vi "关键参数交互.vi"(9 "量程选择":enum16{"低量程", "高量程"}(ring), 11 "模型":enum32{"线性", "多项式", "折线"}(ring)) -> ()   [LabVIEW 2016, in "斯坦道CODMn.lvlib"]
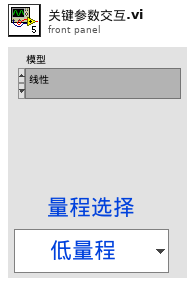
[diagram p1: front panel]
types:
  T1 = cluster{"chose":string, "公式":cluster{"X^2":dbl, "X":dbl, "b":dbl}}
  T2 = cluster{"测量量程":dbl, "测量精度":dbl, "测量间隔":dbl, "消解温度":dbl, "消解时长":dbl, "空白校准时间":timestamp, "曲线截距":dbl, "曲线斜率":dbl, "测量检出限":dbl, "测量信号值":dbl, "线性相关系数":dbl, "二次多项式系数":dbl, "标样校准时间":timestamp, "稀释倍数":dbl, "三项式系数":dbl, "空白标定系数":dbl, "量程系数":dbl, "F0/ORPA":dbl, "F1/ORPB":dbl, "F2/ORPK":dbl, "F3":dbl, "F4":dbl, "F5":dbl, "F6":dbl, "F7":dbl, "X0/滴定数":dbl, "量程":dbl}
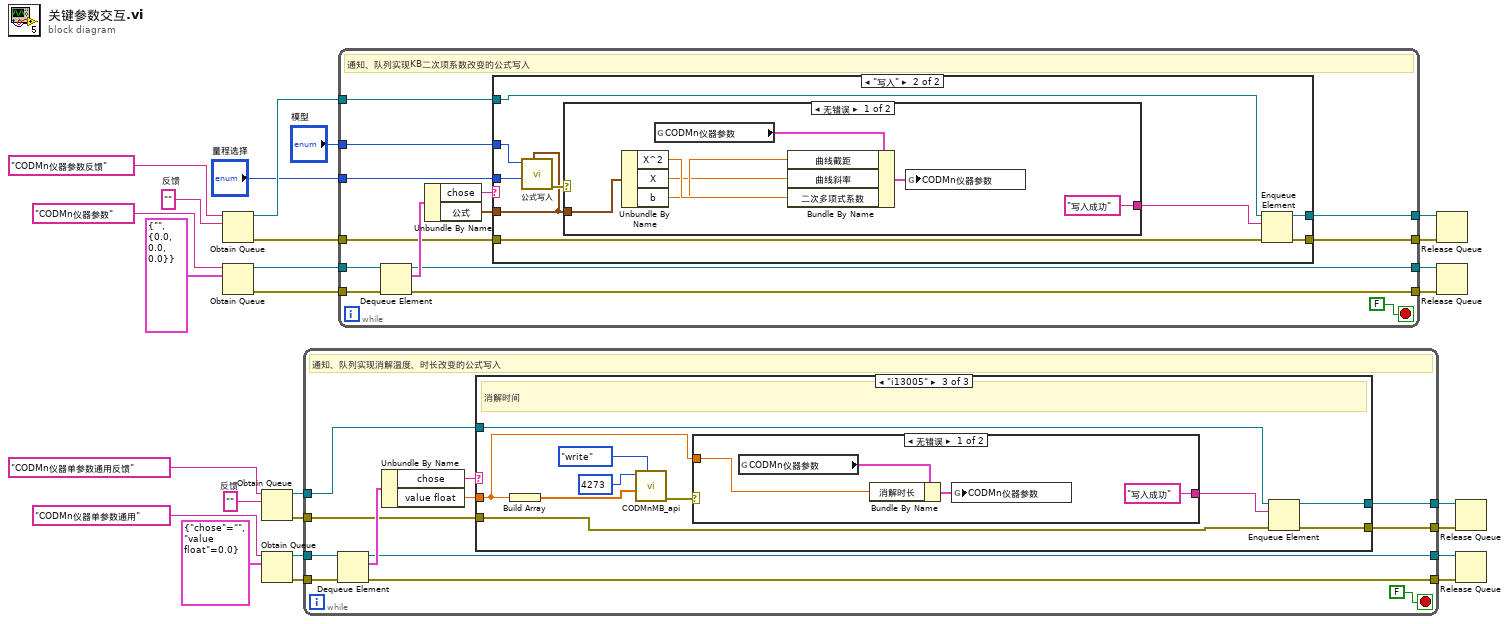
[diagram p0: block diagram]
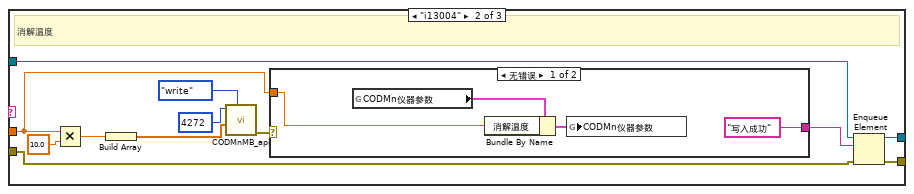
[diagram p3: hidden frame]
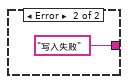
[diagram p4: hidden frame]
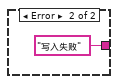
[diagram p5: hidden frame]
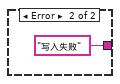
[diagram p7: hidden frame]
diagram:
  w9 = ""  # 反馈
  w18 = ""  # 反馈
  n1 = Obtain Queue(name (unnamed)="CODMn仪器参数反馈" ("名称（未命名）"), element data type=w18) -> (queue out=w19:refnum<queue>, error out=w17:errorcluster)  [unwired: 3 in, 1 out]
  n2 = Obtain Queue(name (unnamed)="CODMn仪器参数" ("名称（未命名）"), element data type=T1 {"chose"="", "公式"={"X^2"=0.0, "X"=0.0, "b"=0.0}}) -> (queue out=w26:refnum<queue>, error out=w25:errorcluster)  [unwired: 3 in, 1 out]
  n3 = Obtain Queue(name (unnamed)="CODMn仪器单参数通用反馈" ("名称（未命名）"), element data type=w9) -> (queue out=w8:refnum<queue>, error out=w10:errorcluster)  [unwired: 3 in, 1 out]
  n4 = Obtain Queue(name (unnamed)="CODMn仪器单参数通用" ("名称（未命名）"), element data type=cluster{"chose":string, "value float":dbl} {"chose"="", "value float"=0.0}) -> (queue out=w1:refnum<queue>, error out=w2:errorcluster)  [unwired: 3 in, 1 out]
  n5 = while {
    tunnel: w1 -> [w37]
    tunnel: w2 -> [w36]
    tunnel: [w32] -> w5
    tunnel: [w31] -> w6
    tunnel: w8 -> [w30]
    tunnel: w10 -> [w29]
    tunnel: [w28] -> w11
    tunnel: [w27] -> w12
    stop <- FALSE stop-if-true
    # "通知、队列实现消解温度、时长改变的公式写入"
    n6 = Dequeue Element(queue=w37, error in (no error)=w36) -> (queue out=w32:refnum<queue>, element=w35:cluster{"chose":string, "value float":dbl}, error out=w31:errorcluster)  [unwired: 1 in, 1 out]
    n7 = Unbundle By Name(w35) -> ("chose"=w34:string, "value float"=w33:dbl)
    n8 = case shown="\"i13005\"" w34 {
      tunnel: w33 -> [_ w41 w58]
      tunnel: w30 -> [w40 w52 w67]
      tunnel: w29 -> [w39 w50 w63]
      tunnel: [w40 w49 w65] -> w28
      tunnel: [w39 w48 w64] -> w27
      frame "假", Default {
      }
      frame "i13004" {
        # "消解温度"
        n9 = Multiply(x=w41, y=10.0) -> (x*y=w44:dbl)
        n10 = Build Array(w44) -> (w43:dbl[])
        n11 = call "CODMnMB_api.vi"("STEP"=enum16{"open", "read", "write", "close"}."write", "values"=w43, "starting address"=u16 4272) -> ("error out"=w42:errorcluster)  [unwired: 6 in, 2 out]
        n12 = case shown="无错误" w42 {
          tunnel: ["写入成功" ("消息") "写入失败" ("消息")] -> w51
          tunnel: w41 -> [w53 _]
          frame No Error {
            n13 = global read "CODMn断电保存全局变量.vi" "CODMn仪器参数"() -> (w55:T2)
            n14 = Bundle By Name(cluster=w55, "消解温度"=w53) -> (w54:T2)
            n15 = global write "CODMn断电保存全局变量.vi" "CODMn仪器参数"(w54) -> ()
          }
          frame Error {
          }
        }
        n16 = Enqueue Element(queue=w52, element=w51, error in (no error)=w50) -> (queue out=w49:refnum<queue>, error out=w48:errorcluster)  [unwired: 1 in, 1 out]
      }
      frame "i13005" {
        # "消解时间"
        n17 = Build Array(w58) -> (w60:dbl[])
        n18 = call "CODMnMB_api.vi"("STEP"=enum16{"open", "read", "write", "close"}."write", "values"=w60, "starting address"=u16 4273) -> ("error out"=w59:errorcluster)  [unwired: 6 in, 2 out]
        n19 = case shown="无错误" w59 {
          tunnel: ["写入成功" ("消息") "写入失败" ("消息")] -> w66
          tunnel: w58 -> [w69 _]
          frame No Error {
            n20 = global read "CODMn断电保存全局变量.vi" "CODMn仪器参数"() -> (w70:T2)
            n21 = Bundle By Name(cluster=w70, "消解时长"=w69) -> (w68:T2)
            n22 = global write "CODMn断电保存全局变量.vi" "CODMn仪器参数"(w68) -> ()
          }
          frame Error {
          }
        }
        n23 = Enqueue Element(queue=w67, element=w66, error in (no error)=w63) -> (queue out=w65:refnum<queue>, error out=w64:errorcluster)  [unwired: 1 in, 1 out]
      }
    }
  }
  n24 = while {
    tunnel: w26 -> [w85]
    tunnel: w25 -> [w84]
    tunnel: [w80] -> w22
    tunnel: [w79] -> w21
    tunnel: w19 -> [w78]
    tunnel: w17 -> [w77]
    tunnel: [w76] -> w16
    tunnel: [w75] -> w15
    tunnel: "模型" -> [w74]
    tunnel: "量程选择" -> [w73]
    stop <- FALSE stop-if-true
    # "通知、队列实现KB二次项系数改变的公式写入"
    n25 = Dequeue Element(queue=w85, error in (no error)=w84) -> (queue out=w80:refnum<queue>, element=w83:T1, error out=w79:errorcluster)  [unwired: 1 in, 1 out]
    n26 = Unbundle By Name(w83) -> ("chose"=w82:string, "公式"=w81:cluster{"X^2":dbl, "X":dbl, "b":dbl})
    n27 = case shown="\"写入\"" w82 {
      tunnel: w81 -> [_ w90]
      tunnel: w78 -> [w88 w97]
      tunnel: w77 -> [w87 w95]
      tunnel: [w88 w94] -> w76
      tunnel: [w87 w93] -> w75
      tunnel: w74 -> [_ w91]
      tunnel: w73 -> [_ w89]
      frame "假", Default {
      }
      frame "写入" {
        n28 = call "公式写入.vi"("公式"=w90, "量程选择"=w89, "模型"=w91) -> ("error out"=w92:errorcluster)  [unwired: 8 in]
        n29 = case shown="无错误" w92 {
          tunnel: ["写入成功" ("消息") "写入失败" ("消息")] -> w96
          tunnel: w90 -> [w98 _]
          frame No Error {
            n30 = Unbundle By Name(w98) -> ("X^2"=w101:dbl, "X"=w99:dbl, "b"=w100:dbl)
            n31 = global read "CODMn断电保存全局变量.vi" "CODMn仪器参数"() -> (w102:T2)
            n32 = Bundle By Name(cluster=w102, "曲线截距"=w100, "曲线斜率"=w99, "二次多项式系数"=w101) -> (w103:T2)
            n33 = global write "CODMn断电保存全局变量.vi" "CODMn仪器参数"(w103) -> ()
          }
          frame Error {
          }
        }
        n34 = Enqueue Element(queue=w97, element=w96, error in (no error)=w95) -> (queue out=w94:refnum<queue>, error out=w93:errorcluster)  [unwired: 1 in, 1 out]
      }
    }
  }
  n35 = Release Queue(queue=w16, error in (no error)=w15) -> ()  [unwired: 1 in, 3 out]
  n36 = Release Queue(queue=w22, error in (no error)=w21) -> ()  [unwired: 1 in, 3 out]
  n37 = Release Queue(queue=w11, error in (no error)=w12) -> ()  [unwired: 1 in, 3 out]
  n38 = Release Queue(queue=w5, error in (no error)=w6) -> ()  [unwired: 1 in, 3 out]
